vi "Remove Controls from Selection.vi"(8 "Error In":errorcluster) -> (0 "Error Out":errorcluster)   [LabVIEW 2018, in "Toolkit.lvlib" / "Tests.lvlib"]
uses:
  Tests.lvlib
  <vilib>/Utility/traverseref.llb/TRef TravTarget.ctl
  <vilib>/addons/_JKI Toolkits/Caraya/classes/Test/Test.lvclass
  <vilib>/Utility/traverseref.llb/VI Scripting - Traverse.lvlib
  <vilib>/addons/_JKI Toolkits/Caraya/classes/Assert/Assert.lvclass
  Toolkit.lvlib
  tests/Tests.lvlib
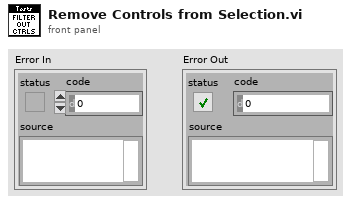
[diagram p1: front panel]
types:
  T1 = typedef "TRef TravTarget.ctl" = enum16{"FP", "BD", "Other"}
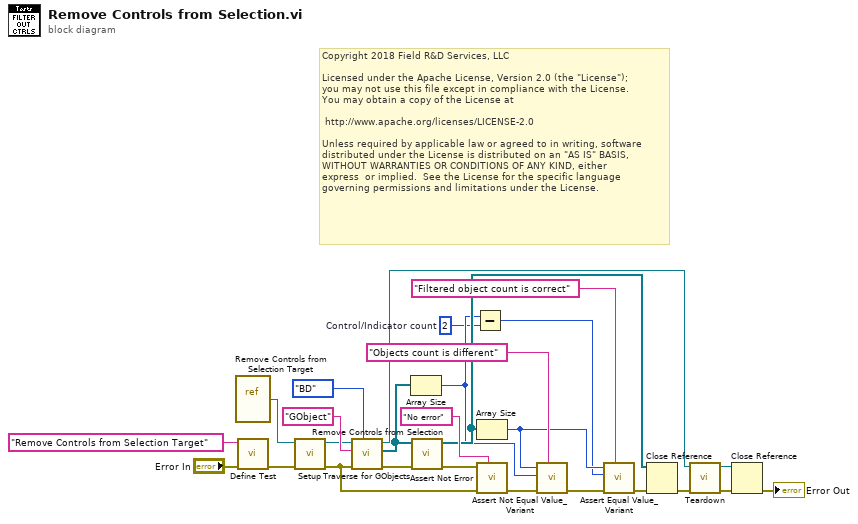
[diagram p0: block diagram]
diagram:
  w2 = 2  # Control/Indicator count
  # "Copyright 2018 Field R&D Services, LLC\n\nLicensed under the Apache License, Version 2.0 (the \"License\");\nyou may not use this file except in compliance with the License.\nYou may obtain a copy of the License at\n\n\thttp://www.apache.org/licenses/LICENSE-2.0\n\nUnless required by applicable law or agreed to in writing, software\ndistributed under the License is distributed on an \"AS IS\" BASIS,\nWITHOUT WARRANTIES OR CONDITIONS OF ANY KIND, either \nexpress  or implied.  See the License for the specific language \ngoverning permissions and limitations under the License."
  n1 = vi-ref "Remove Controls from Selection Target.vi"() -> (w23:refnum<vi>)
  n2 = call <vilib>:"Define Test.vi"("error in (no error)"="Error In", "Label (VI Title)"="Remove Controls from Selection Target") -> ("error out"=w17:errorcluster)  [unwired: 9 in]
  n3 = call "Setup.vi"("Error In"=w17, "VI In"=w23) -> ("Error Out"=w15:errorcluster, "VI Out"=w22:refnum<vi>)  [unwired: 8 in]
  n4 = call <vilib>:"Traverse for GObjects.vi"("Traverse Target"=TRef_TravTarget."BD", "error in (no error)"=w15, "Class Name"="GObject", "VI Refnum"=w22) -> ("error out"=w24:errorcluster, "References"=w7:refnum<vi>[], "dup VI Refnum"=w21:refnum<vi>)  [unwired: 4 in, 1 out]
  n5 = Array Size(array=w7) -> (size(s)=w3:i32)
  n6 = call "Remove Controls from Selection.vi"("Error In"=w24, "Selection"=w7) -> ("Error Out"=w13:errorcluster, "Filtered Selection"=w8:refnum<vi>[])  [unwired: 8 in]
  n7 = Subtract(x=w3, y=w2) -> (x-y=w1:i32)
  n8 = Array Size(array=w8) -> (size(s)=w5:i32)
  n9 = call <vilib>:"Assert Not Error.vi"("Label"="No error", "error in (no error)"=w15, "Not Error?"=w13) -> ("error out"=w14:errorcluster)  [unwired: 8 in]
  n10 = call <vilib>:"Assert Not Equal Value_Variant.vi"("Label"="Objects count is different", "error in (no error)"=w14, "Y"=w3, "X"=w5) -> ("error out"=w10:errorcluster)  [unwired: 7 in]
  n11 = call <vilib>:"Assert Equal Value_Variant.vi"("Label"="Filtered object count is correct", "error in (no error)"=w10, "Y"=w1, "X"=w5) -> ("error out"=w6:errorcluster)  [unwired: 7 in]
  n12 = Close Reference(reference=w8, error in (no error)=w6) -> (error out=w9:errorcluster)
  n13 = call "Teardown.vi"("Error In"=w9, "VI In"=w21) -> ("Error Out"=w19:errorcluster, "VI Out"=w20:refnum<vi>)  [unwired: 8 in]
  n14 = Close Reference(reference=w20, error in (no error)=w19) -> (error out=→"Error Out":errorcluster)
